vi "Set IConfigurationStrategy.vi"(10 "IConfigurationStrategy":refnum<class "IConfigurationStrategy.lvclass">, 11 "NI 9862 in":refnum<class "NI 9862.lvclass">) -> (3 "NI 9862 out":refnum<class "NI 9862.lvclass">)   [LabVIEW 2024, in "NI 9862.lvclass"]
uses:
  NI 9862.lvclass
  NI 9862.lvclass/NI 9862.ctl
  Source/Interfaces/IConfigurationStrategy/IConfigurationStrategy.lvclass
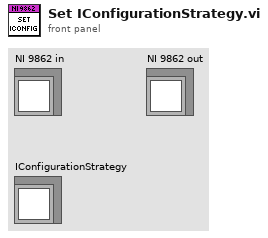
[diagram p1: front panel]
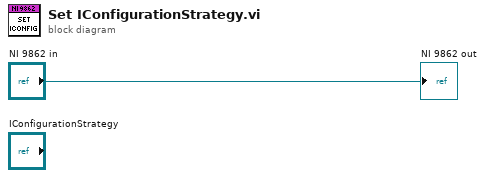
[diagram p0: block diagram]
diagram:
  "NI 9862 out" <- "NI 9862 in"
